vi "Actor Core.vi"(8 "error in":errorcluster, 11 "App in":refnum<class "App.lvclass">) -> (0 "error out":errorcluster, 3 "Actor out":refnum<class "Actor.lvclass">)   [LabVIEW 2016, in "App.lvlib" / "App.lvclass"]
doc: "(<B>Filename</B>: Actor Framework.lvlib:Actor.lvclass:Actor Core.vi)\n\nReceives messages to the actor, reacts to them, and initiates any error handling that may shut the actor down.\n\nDescendant classes may override this VI to append parallel tasks for the actor to complete while it handles messages. Overrides use the Call Parent Method node."
uses:
  App.lvclass
  C:/Program Files/National Instruments/LabVIEW 2016/vi.lib/ActorFramework/Actor/Actor.lvclass
  <vilib>/ActorFramework/Actor/Actor.lvclass
  App.lvclass/App.ctl
  Dynamic Instrument/Dynamic Instrument/Dynamic Instrument.lvclass/Dynamic Instrument.ctl
  <vilib>/ActorFramework/Actor/Actor.lvclass/Actor.ctl
  <vilib>/ActorFramework/Message Enqueuer/Message Enqueuer.lvclass/Message Enqueuer.ctl
  Dynamic Instrument/Dynamic Instrument/Read Instrument Name.vi
  <vilib>/ActorFramework/Message Enqueuer/Init from Existing Queue.vi
  <vilib>/ActorFramework/Message Enqueuer/Enqueue.vi
  <vilib>/ActorFramework/Stop Msg/Stop Msg.lvclass
  C:/Program Files/National Instruments/LabVIEW 2016/vi.lib/ActorFramework/Message/Message.lvclass
  <vilib>/ActorFramework/Message Priority Queue/Priority Enqueue.vi
  <vilib>/ActorFramework/Message Enqueuer/Message Enqueuer.lvclass
  Dynamic Instrument/Dynamic Instrument/Dynamic Instrument.lvclass
panel:
  out "Application:Name":string
  out "Load Path":path
  out "Instruments":string[](array[string])
  out "DAQmx loaded":bool
  in  "Stop Button":bool
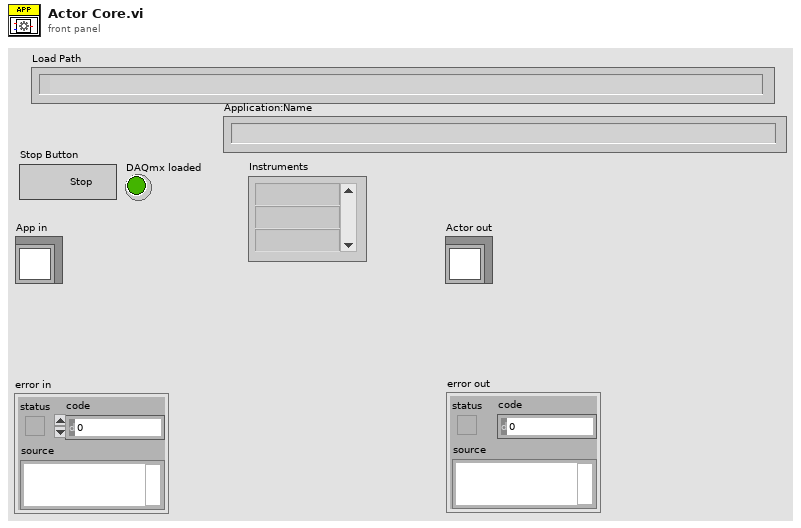
[diagram p1: front panel]
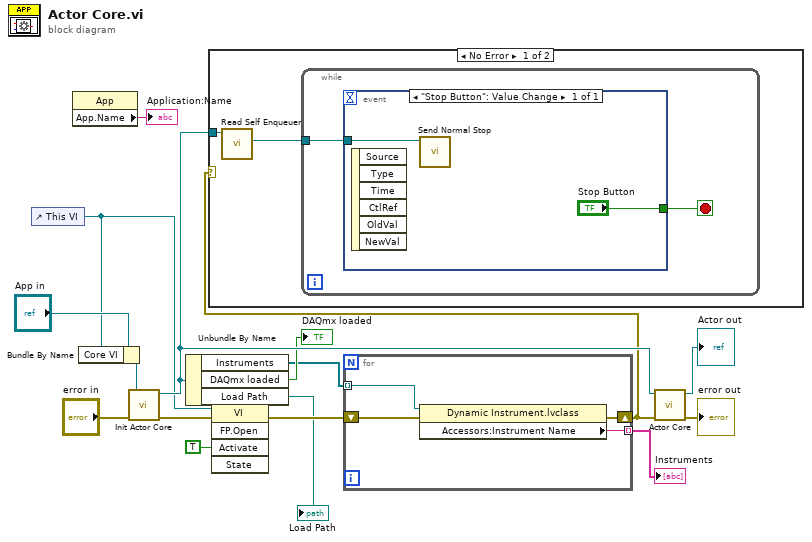
[diagram p0: block diagram]
diagram:
  n1 = control-ref of="This VI"() -> (w4:refnum<vi>)
  n2 = property class="App"() -> ("App.Name"=→"Application:Name":string)  [unwired: 2 in, 2 out]
  n3 = Bundle By Name(cluster="App in", "Core VI"=w4) -> (w5:refnum<class "App.lvclass">)
  n4 = call-dynamic "Init Actor Core.vi"("error in (no error)"="error in", "App in"=w5) -> ("error out"=w7:errorcluster, "App out"=w12:refnum<class "App.lvclass">)  [unwired: 8 in]
  n5 = Unbundle By Name(w12) -> ("Instruments"=w10:refnum<class "Dynamic Instrument.lvclass">[], "DAQmx loaded"=→"DAQmx loaded":bool, "Load Path"=→"Load Path":path)
  n6 = invoke class="VI" method="FP.Open"(reference=w4, error in=w7, "Activate"=TRUE ("Activate?")) -> (error out=w6:errorcluster)  [unwired: 2 in, 4 out]
  n7 = for {
    tunnel: w10 -> [w20] mode=indexing
    tunnel: [w19] -> w9 mode=indexing
    shift-right: [w17] -> w2
    shift-left: w6 -> [w18]
    n8 = property class="Dynamic Instrument.lvclass"(reference=w20, error in=w18) -> (error out=w17:errorcluster, "Accessors:Instrument Name"=w19:string)  [unwired: 1 out]
  }
  "Instruments" <- w9
  n9 = case shown="No Error" w2 {
    tunnel: w12 -> [w21 _]
    frame No Error {
      n10 = call <vilib>:"Read Self Enqueuer.vi"("Actor"=w21) -> ("Self Enqueuer"=w22:refnum<class "Message Enqueuer.lvclass">)  [unwired: 10 in]
      n11 = while {
        tunnel: w22 -> [w23]
        stop <- w24 stop-if-true
        n12 = event shown="[0] \"Stop Button\": Value Change" {
          selector: _ -> [_]
          dyn-events: _ -> [_]
          timeout: _ -> [_]
          tunnel: ["Stop Button"] -> w24
          tunnel: w23 -> [w25]
          event "Stop Button": Value Change {
            n13 = event-data() -> ()  [unwired: 1 in, 6 out]
            n14 = call <vilib>:"Send Normal Stop.vi"("Message Enqueuer"=w25) -> ()  [unwired: 10 in, 1 out]
          }
        }
      }
    }
    frame Error {
    }
  }
  n15 = call-parent "Actor Core.vi"("error in"=w2, "Actor in"=w12) -> ("error out"=→"error out":errorcluster, "Actor out"=→"Actor out":refnum<class "Actor.lvclass">)  [unwired: 8 in]
